vi "Construct.vi"(1 "Parent":refnum<vi>, 2 "Has Parent":bool, 3 "Local Position":refnum<class "Vector2.lvclass">) -> (0 "Transform out":refnum<class "Transform.lvclass">)   [LabVIEW 2022 SP3, in "Transform.lvclass"]
uses:
  Transform.lvclass
  Math/Vector2/Vector2.lvclass
  Transform.lvclass/Transform.ctl
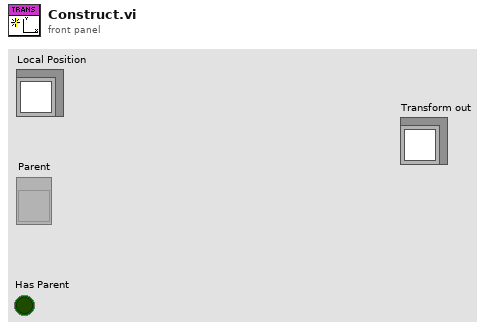
[diagram p1: front panel]
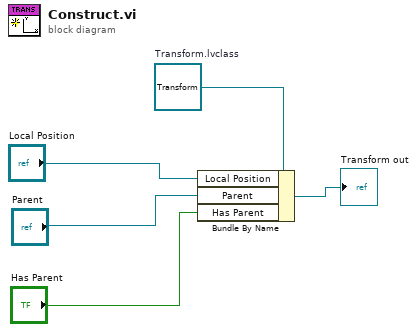
[diagram p0: block diagram]
diagram:
  w5 = refnum<class "Transform.lvclass"> refnum  # Transform.lvclass
  n1 = Bundle By Name(cluster=w5, "Local Position"="Local Position", "Parent"="Parent", "Has Parent"="Has Parent") -> (→"Transform out":refnum<class "Transform.lvclass">)
